vi "Read Path to check.vi"(11 "CDependencyInspection in":refnum<class "CDependencyInspection.lvclass">) -> (2 "Path to check":path, 3 "CDependencyInspection out":refnum<class "CDependencyInspection.lvclass">)   [LabVIEW 2020, in "DependencyInspection.lvlib" / "CDependencyInspection.lvclass"]
uses:
  CDependencyInspection.lvclass
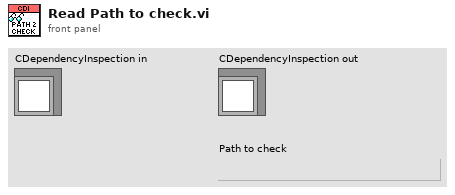
[diagram p1: front panel]
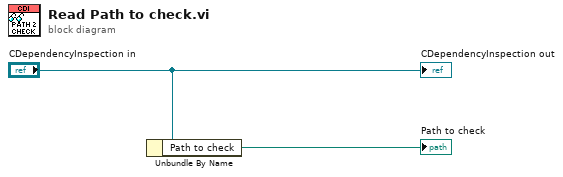
[diagram p0: block diagram]
diagram:
  n1 = Unbundle By Name("CDependencyInspection in") -> ("Path to check"=→"Path to check":path)
  "CDependencyInspection out" <- "CDependencyInspection in"
